vi "String Value.vi"(1 "Length":i32, 2 "Offset":string, 3 "string":string) -> (0 "Value":string)   [LabVIEW 2012]
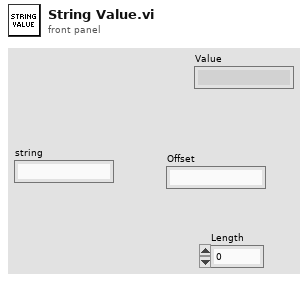
[diagram p1: front panel]
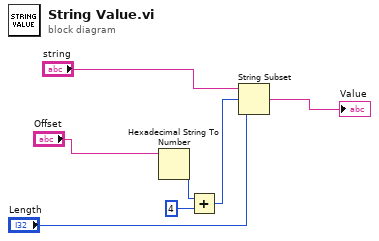
[diagram p0: block diagram]
diagram:
  n1 = Hexadecimal String To Number(string="Offset") -> (number=w5:u32)  [unwired: 2 in, 1 out]
  n2 = Add(x=w5, y=u32 4) -> (x+y=w3:u32)
  n3 = String Subset(string="string", offset (0)=w3, length (rest)="Length") -> (substring=→"Value":string)
